vi "Create Sessions - 1Sess.vi"(6 "initialize and close session behavior":T1, 7 "option string":string, 8 "error in":errorcluster, 9 "reset":bool, 11 "session reservation in":refnum<class "Session Reservation.lvclass">) -> (0 "error out":errorcluster, 1 "channel list":string, 2 "session":refnum<k15>, 3 "session reservation out":refnum<class "Session Reservation.lvclass">)   [LabVIEW 2020, in "MeasurementLink niScope.lvlib"]
doc: "Create the NI-SCOPE driver session from the <b>session reservation in</b>. Returns an error if more than one NI-SCOPE session has been reserved. Use \"Create Session - NSess.vi\" for multiple sessions."
uses:
  MeasurementLink niScope.lvlib
  MeasurementLink Session Management/Session Reservation/Session Reservation.lvclass
  081d95db-f041-4b50-9562-e62bb01ed17a.vi
  Instrument/Instrument.lvclass
  \\tsclient\C/dev/measurementlink-labview/Source/Runtime/MeasurementLink Instrument/IInstrument/IInstrument.lvclass
  MeasurementLink Session Management/Session Reservation/Create Sessions Impl.vi
  MeasurementLink Session Management/Session Reservation/Initialize and Close Session Behavior.ctl
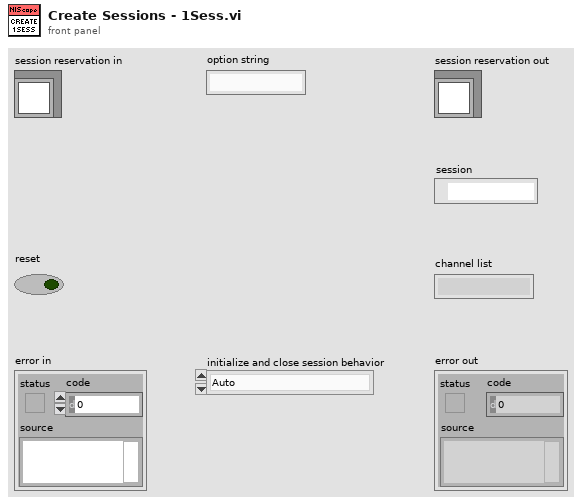
[diagram p1: front panel]
types:
  T1 = typedef "MeasurementLink Session Management.lvlib/Session Reservation.lvclass/Initialize and Close Session Behavior.ctl" = enum16{"Auto", "Create and Close", "Attach and Detach", "Create and Detach", "Attach and Close"}
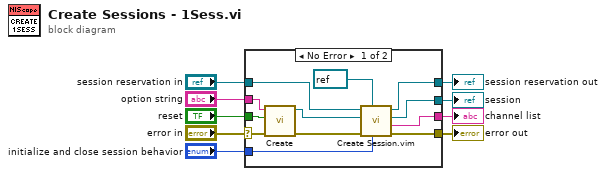
[diagram p0: block diagram]
diagram:
  n1 = case shown="No Error" "error in" {
    selector: "error in" -> [w20 w23]
    tunnel: [w17 w23] -> w8
    tunnel: [w21 w22] -> w6
    tunnel: "session reservation in" -> [w14 w22]
    tunnel: "option string" -> [w18 _]
    tunnel: "reset" -> [w19 _]
    tunnel: [w16 _] -> w3
    tunnel: [w11 _] -> w2
    tunnel: "initialize and close session behavior" -> [w10 _]
    frame No Error {
      n2 = call "Create.vi"("error in"=w20, "reset"=w19, "option string"=w18) -> ("error out"=w13:errorcluster, "instrument out"=w15:refnum<class "Instrument.lvclass">)  [unwired: 7 in]
      n3 = call "Create Session.vim"("initialize and close session behavior"=w10, "session type"=refnum<k15> refnum ("instrument handle out"), "error in"=w13, "instrument"=w15, "session reservation in"=w14) -> ("error out"=w17:errorcluster, "channel list"=w16:string, "session"=w11:refnum<k15>, "session reservation out"=w21:refnum<class "Session Reservation.lvclass">)  [unwired: 3 in]
    }
    frame Error {
    }
  }
  "error out" <- w8
  "session reservation out" <- w6
  "channel list" <- w3
  "session" <- w2
